vi "VeriStand DSF.Transfer.Configuration.Get Device Reference.vi"(11 "VeriStand DSF.Transfer.Configuration in":refnum<class "VeriStand DSF.Transfer.Configuration.lvclass">) -> (2 "Device Reference":T1=18446744073709551615 format="%.0x", 3 "VeriStand DSF.Transfer.Configuration out":refnum<class "VeriStand DSF.Transfer.Configuration.lvclass">)   [LabVIEW 2017, in "Data Sharing Framework Engine.lvlib" / "VeriStand DSF.Transfer.Configuration.lvclass"]
uses:
  VeriStand DSF.Transfer.Configuration.lvclass
  <vilib>/NI Veristand/Custom Device API/Custom Device Item Ref.ctl
  VeriStand DSF.Transfer.Configuration.lvclass/VeriStand DSF.Transfer.Configuration.ctl
  <vilib>/NI Veristand/Custom Device API/Custom Device API.lvlib
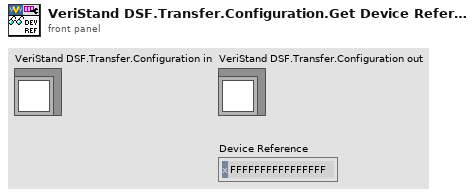
[diagram p1: front panel]
types:
  T1 = typedef "Custom Device API.lvlib/Custom Device Item Ref.ctl" = u64
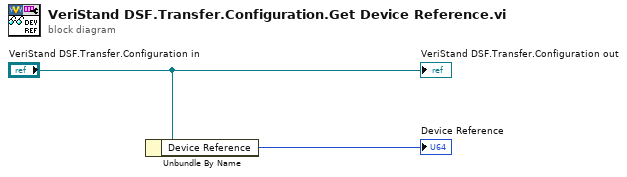
[diagram p0: block diagram]
diagram:
  n1 = Unbundle By Name("VeriStand DSF.Transfer.Configuration in") -> ("Device Reference"=→"Device Reference":T1)
  "VeriStand DSF.Transfer.Configuration out" <- "VeriStand DSF.Transfer.Configuration in"
